vi "Smart Open VI Locaiton.vi"(6 "Variant in":variant, 7 "Shift Pressed?":bool, 8 "error in (no error)":errorcluster, 10 "QD Combo Box Ref":refnum<vi>, 11 "QD Launch VI Ref":refnum<vi>) -> (0 "error out":errorcluster, 4 "Variant out":variant)   [LabVIEW 2012, in "Smart Open VI Location.lvlib"]
doc: "When triggered on Front Panel:\nOpen Current VI's Location in Explorer Window.\n\nWhen triggered on Block Diagram:\nNo SubVI is selected: Open Current VI's Location in Explorer Window.\nSubVIs are selected: Open Selected VI's Location in Explorer Window.\n\nDefault Shortcut - [O]"
uses:
  Smart Open VI Location.lvlib
panel:
  in  "Undo Name":string="Quick Drop Keyboard Shortcut"
  # "Do not change the connector pane of this VI.\n\nSee the block diagram for directions on how to use this template."
  # "Specify the name of the Undo transaction"
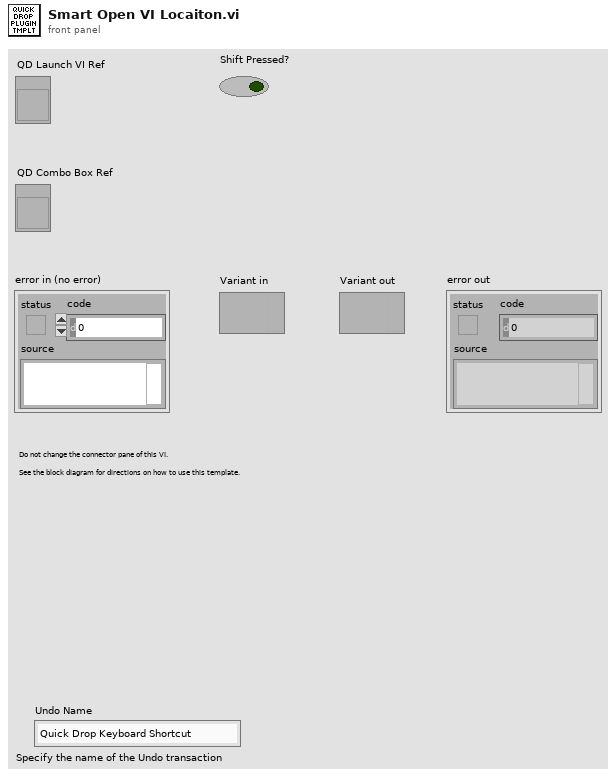
[diagram p1: front panel]
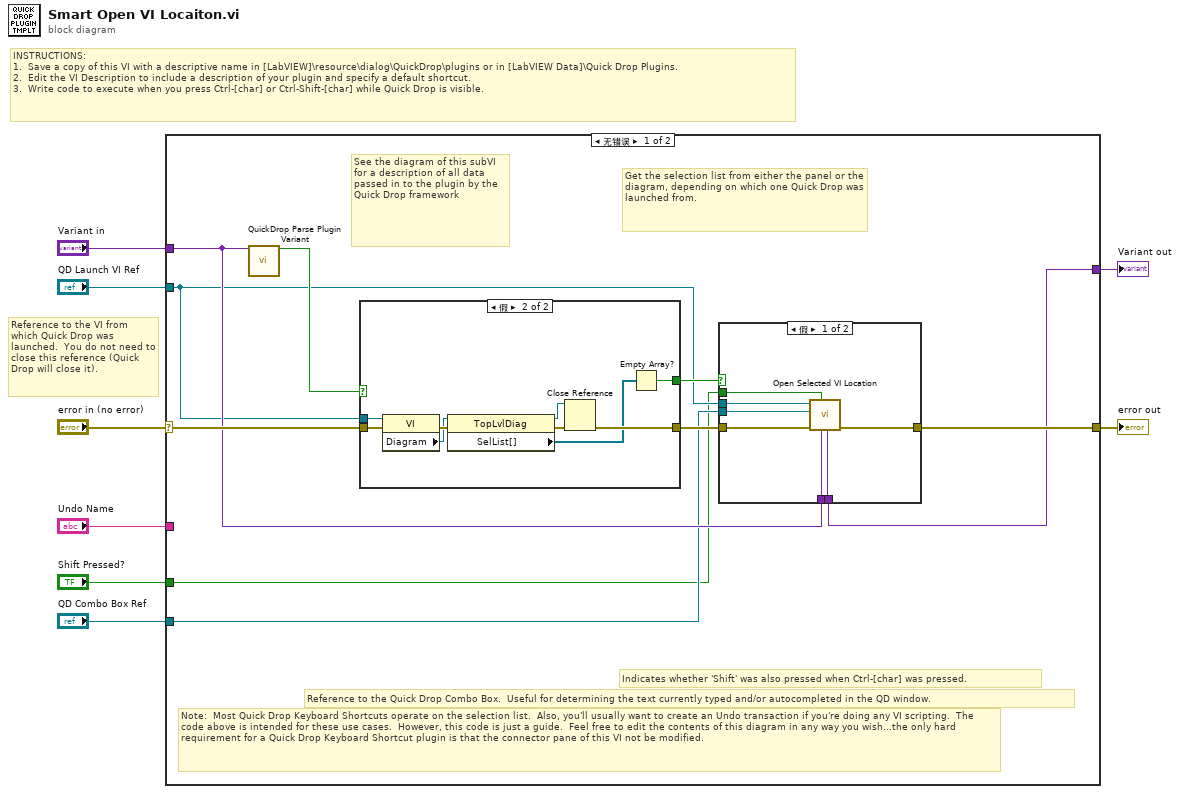
[diagram p0: block diagram]
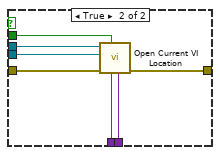
[diagram p2: hidden frame]
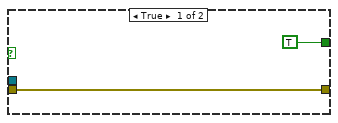
[diagram p3: hidden frame]
diagram:
  # "Reference to the VI from which Quick Drop was launched.  You do not need to close this reference (Quick Drop will close it)."
  # "INSTRUCTIONS:\n1.  Save a copy of this VI with a descriptive name in [LabVIEW]\\resource\\dialog\\QuickDrop\\plugins or in [LabVIEW Data]\\Quick Drop Plugins.\n2.  Edit the VI Description to include a description of your plugin and specify a default shortcut. \n3.  Write code to execute when you press Ctrl-[char] or Ctrl-Shift-[char] while Quick Drop is visible."
  n1 = case shown="无错误" "error in (no error)" {
    selector: "error in (no error)" -> [w18 w44]
    tunnel: [w14 w44] -> w7
    tunnel: "QD Launch VI Ref" -> [w10 _]
    tunnel: "Shift Pressed?" -> [w9 _]
    tunnel: "QD Combo Box Ref" -> [w11 _]
    tunnel: "Variant in" -> [w13 _]
    tunnel: "Undo Name" -> [_ _]
    tunnel: [w12 _] -> w1
    frame No Error {
      # "Note:  Most Quick Drop Keyboard Shortcuts operate on the selection list.  Also, you'll usually want to create an Undo transaction if you're doing any VI scripting.  The code above is intended for these use cases.  However, this code is just a guide.  Feel free to edit the contents of this diagram in any way you wish...the only hard requirement for a Quick Drop Keyboard Shortcut plugin is that the connector pane of this VI not be modified."
      # "Get the selection list from either the panel or the diagram, depending on which one Quick Drop was launched from."
      # "See the diagram of this subVI for a description of all data passed in to the plugin by the Quick Drop framework"
      # "Reference to the Quick Drop Combo Box.  Useful for determining the text currently typed and/or autocompleted in the QD window."
      # "Indicates whether 'Shift' was also pressed when Ctrl-[char] was pressed."
      n2 = call <vilib>:"QuickDrop Parse Plugin Variant.vi"("QDKS Variant in"=w13) -> ("QD Launch VI Panel?"=w17:bool)  [unwired: 12 in, 2 out]
      n3 = case shown="假" w17 {
        tunnel: w18 -> [w34 w43]
        tunnel: w10 -> [_ w42]
        tunnel: [w34 w37] -> w15
        tunnel: [TRUE w36] -> w16
        frame True {
        }
        frame False {
          n4 = property class="VI"(reference=w42, error in=w43) -> (error out=w41:errorcluster, "Diagram"=w40:refnum<vi>)  [unwired: 1 out]
          n5 = property class="TopLvlDiag"(reference=w40, error in=w41) -> (reference out=w38:refnum<vi>, error out=w39:errorcluster, "SelList[]"=w35:refnum<vi>[])
          n6 = Close Reference(reference=w38, error in (no error)=w39) -> (error out=w37:errorcluster)
          n7 = Empty Array?(array=w35) -> (empty?=w36:bool)
        }
      }
      n8 = case shown="假" w16 {
        tunnel: w15 -> [w25 w32]
        tunnel: [w24 w31] -> w14
        tunnel: w13 -> [w23 w30]
        tunnel: [w22 w29] -> w12
        tunnel: w11 -> [w20 w28]
        tunnel: w10 -> [w21 w27]
        tunnel: w9 -> [w19 w26]
        frame False {
          n9 = call "Open Selected VI Location.vi"("Variant in"=w23, "Shift Pressed?"=w19, "error in (no error)"=w25, "QD Combo Box Ref"=w20, "QD Launch VI Ref"=w21) -> ("error out"=w24:errorcluster, "Variant out"=w22:variant)  [unwired: 5 in]
        }
        frame True {
          n10 = call "Open Current VI Location.vi"("Variant in"=w30, "Shift Pressed?"=w26, "error in (no error)"=w32, "QD Combo Box Ref"=w28, "QD Launch VI Ref"=w27) -> ("error out"=w31:errorcluster, "Variant out"=w29:variant)  [unwired: 5 in]
        }
      }
    }
    frame Error {
    }
  }
  "error out" <- w7
  "Variant out" <- w1
